vi "Constants.vi"() -> ()   [LabVIEW 2013, in "Trigger Timestamp Logging Shared.lvlib"]
doc: "Use this Global VI to access the GUIDs assigned to the page resources of the Custom Device."
uses:
  Trigger Timestamp Logging Shared.lvlib
panel:
  in  "Tab Control":enum32{"GUIDS", "Constants", "Properties"}(tab)
  in  "Trigger Timestamp Logging":string="d84d6791-5164-41fa-918c-66c2e4f1039d"
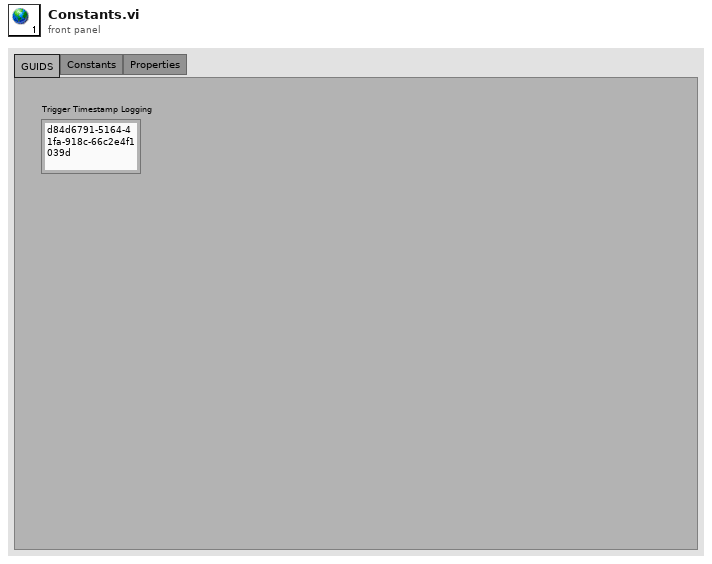
[diagram p1: front panel]
diagram:
